vi "SendMessage_Cluster.vi"(6 "timeout in ms (-1)":i32=-1, 8 "error in":errorcluster, 10 "message":T1, 11 "message ref in":refnum<class "CLM_LocalMessage_UserEvent.lvclass">) -> (0 "error out":errorcluster, 3 "message ref out":refnum<class "CLM_LocalMessage_UserEvent.lvclass">, 4 "timed out?":bool)   [LabVIEW 2013, in "CLM_LocalMessage_UserEvent.lvclass"]
uses:
  CLM_LocalMessage_UserEvent.lvclass
  LocalMessage/Message.ctl
  CLM_LocalMessage_UserEvent.lvclass/CLM_LocalMessage_UserEvent.ctl
  LocalMessage/CLM_LocalMessage.lvclass
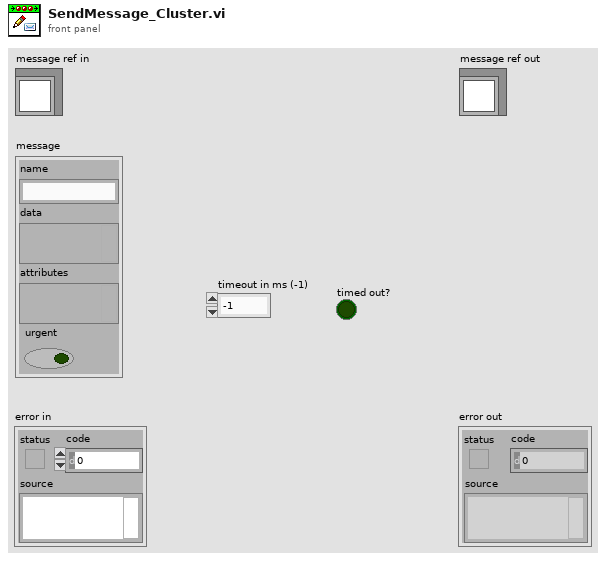
[diagram p1: front panel]
types:
  T1 = typedef "CLM_LocalMessage.lvclass/Message.ctl" = cluster{"name":string, "data":variant, "attributes":variant, "urgent":bool}
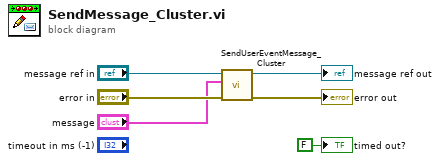
[diagram p0: block diagram]
diagram:
  n1 = call "SendUserEventMessage_Cluster.vi"("error in"="error in", "message"="message", "message ref in"="message ref in") -> ("error out"=→"error out":errorcluster, "message ref out"=→"message ref out":refnum<class "CLM_LocalMessage_UserEvent.lvclass">)  [unwired: 7 in]
  "timed out?" <- FALSE ("timed out?")
